vi "ReadMultipleDigitalOutputs.vi"(8 "error in (no error)":errorcluster, 11 "TesteractHAL_DigitalOutput_EthernetModbus In":refnum<class "TesteractHAL_DigitalOutput_EthernetModbus.lvclass">) -> (0 "error out":errorcluster, 2 "data":bool[](array[boolean]), 3 "TesteractHAL_DigitalOutput_EthernetModbus Out":refnum<class "TesteractHAL_DigitalOutput_EthernetModbus.lvclass">)   [LabVIEW 2017, in "TesteractHAL_DigitalOutput_EthernetModbus.lvlib" / "TesteractHAL_DigitalOutput_EthernetModbus.lvclass"]
uses:
  TesteractHAL_DigitalOutput_EthernetModbus.lvclass
  C:/Program Files (x86)/Testeract/HWLib/HAL/Device/TesteractHAL_Device.lvlibp/TesteractHAL_Device.lvclass
  TesteractHAL_DigitalOutput_EthernetModbus.lvclass/TesteractHAL_DigitalOutput_EthernetModbus.ctl
  Program Files (x86)/Testeract/HWLib/HAL/Device/TesteractHAL_Device.lvlibp/ReadConnectionAlias.vi
  Drivers/NIModbus/NI Modbus.llb/MB Ethernet Master Query Read Coils (poly).vi
  Program Files (x86)/Testeract/TCPConnectionManager/Testeract_TCPConnectionManager.lvlibp/Testeract_TCPConnectionManager.lvclass
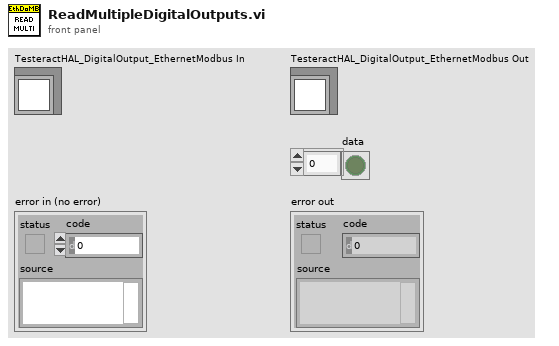
[diagram p1: front panel]
types:
  T1 = typedef "Testeract_TCPConnectionManager.lvlibp/Semaphore RefNum" = refnum<k1>
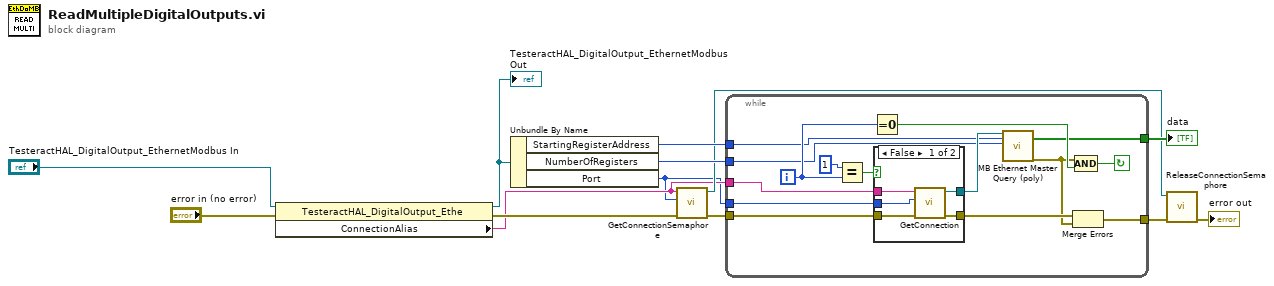
[diagram p0: block diagram]
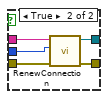
[diagram p2: hidden frame]
diagram:
  n1 = property class="TesteractHAL_DigitalOutput_Ethe"(reference="TesteractHAL_DigitalOutput_EthernetModbus In", error in="error in (no error)") -> (reference out=w8:refnum<class "TesteractHAL_DigitalOutput_EthernetModbus.lvclass">, error out=w5:errorcluster, "ConnectionAlias"=w2:string)
  "TesteractHAL_DigitalOutput_EthernetModbus Out" <- w8
  n2 = Unbundle By Name(w8) -> ("StartingRegisterAddress"=w10:u16, "NumberOfRegisters"=w11:u16, "Port"=w1:u16)
  n3 = call "GetConnectionSemaphore.vi"("error in (no error)"=w5, "Port"=w1, "IPAddress"=w2) -> ("error out"=w4:errorcluster, "Semaphore Ref"=w3:T1)  [unwired: 7 in]
  n4 = while {
    tunnel: w11 -> [w17]
    tunnel: w2 -> [w28]
    tunnel: w4 -> [w27]
    tunnel: [w20] -> w7
    tunnel: [w16] -> w12
    tunnel: w10 -> [w15]
    tunnel: w1 -> [w14]
    i -> [w22]
    stop <- w23 continue-if-true
    n5 = Equal?(x=1, y=w22) -> (x = y?=w25:bool)
    n6 = Equal To 0?(x=w22) -> (x = 0?=w21:bool)
    n7 = case shown="False" w25 {
      tunnel: w28 -> [w30 w35]
      tunnel: w27 -> [w33 w38]
      tunnel: [w31 w36] -> w18
      tunnel: [w32 w37] -> w24
      tunnel: w14 -> [w29 w34]
      frame False {
        n8 = call "GetConnection.vi"("error in (no error)"=w33, "Port"=w29, "IPAddress"=w30) -> ("error out"=w32:errorcluster, "Connection ID"=w31:refnum<k5>)  [unwired: 7 in]
      }
      frame True {
        n9 = call "RenewConnection.vi"("error in (no error)"=w38, "Port"=w34, "IPAddress"=w35) -> ("error out"=w37:errorcluster, "Connection ID"=w36:refnum<k5>)  [unwired: 7 in]
      }
    }
    n10 = call-poly "MB Ethernet Master Query (poly).vi"("TCP Connection Refnum in"=w18, "Starting Address"=w15, "Quantity"=w17) -> ("Coils"=w16:bool[], "error out"=w19:errorcluster)  [unwired: 2 in, 13 out]
    n11 = Merge Errors(w24, w19) -> (w20:errorcluster)
    n12 = Compound Arithmetic op=AND(w19, w21) -> (w23:bool)
  }
  "data" <- w12
  n13 = call "ReleaseConnectionSemaphore.vi"("error in (no error)"=w7, "Semaphore Refnum"=w3) -> ("error out"=→"error out":errorcluster)  [unwired: 9 in]
